vi "Command Tranform.vi"(1 "Command":u16(ring) items=["Move2Pos", "Move2Work", "ChangeManipulator", "Move2Home", "Calibration", "CurrentPos", "Interrupt"]) -> (0 "command str":string)   [LabVIEW 2014]
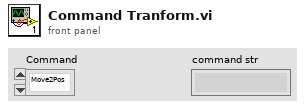
[diagram p1: front panel]
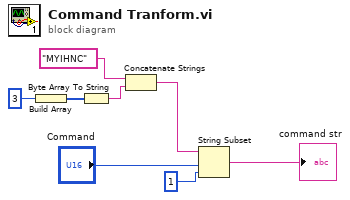
[diagram p0: block diagram]
diagram:
  n1 = Build Array(3) -> (w4:i32[])
  n2 = Byte Array To String(unsigned byte array=w4) -> (string=w6:string)
  n3 = Concatenate Strings("MYIHNC", w6) -> (w8:string)
  n4 = String Subset(string=w8, offset (0)="Command", length (rest)=1 ("length (rest)")) -> (substring=→"command str":string)
